vi "Vector_Plotting.vi"(1 "Template Filename":path, 2 "Data":string[][](array[string]), 3 "Channel Names":string[](array[string])) -> ()   [LabVIEW 2010]
uses:
  Data_File_Type.ctl
  Controls/Group_Binning.ctl
  Globals/Constants_global.vi
panel:
  in  "V":u16(ring) items=["LDA (UW) X Position (mm)", "LDA (UW) Y Position (mm)", "LDA (UW) Z Position (mm)", "Model Mean LDA (U)", "Model Mean LDA (W)"]
  in  "U":u16(ring) items=["LDA (UW) X Position (mm)", "LDA (UW) Y Position (mm)", "LDA (UW) Z Position (mm)", "Model Mean LDA (U)", "Model Mean LDA (W)"]
  in  "Y Axis":u16(ring) items=["LDA (UW) X Position (mm)", "LDA (UW) Y Position (mm)", "LDA (UW) Z Position (mm)", "Model Mean LDA (U)", "Model Mean LDA (W)"]
  in  "X Axis":u16(ring) items=["LDA (UW) X Position (mm)", "LDA (UW) Y Position (mm)", "LDA (UW) Z Position (mm)", "Model Mean LDA (U)", "Model Mean LDA (W)"]
  in  "OK Button":bool
  in  "Row Selector":i32(listbox)=1
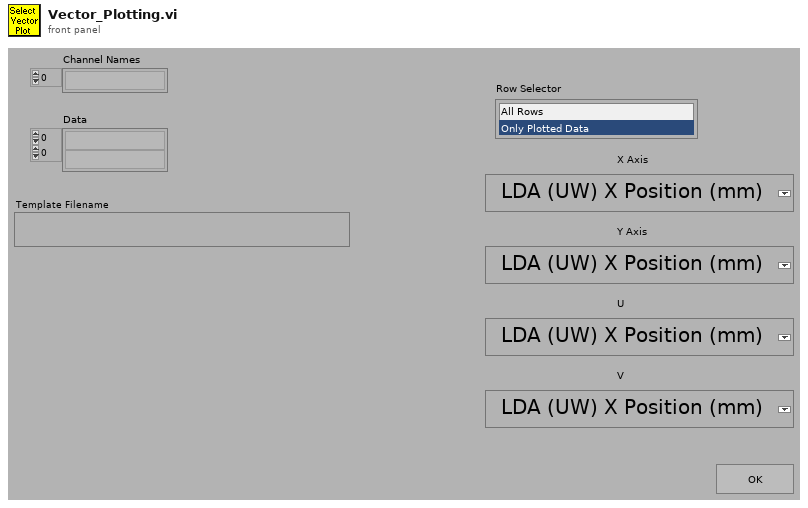
[diagram p1: front panel]
types:
  T1 = typedef "Data_File_Type.ctl" = enum16{"Read All File Types", "Results Files Only", "Raw Data Files Only", "Calibration Files Only", "Gas Desk Files Only", "Old Results Files Only", "Tabulated Data Files Only"}
  T2 = enum16{"Show only data summary", "Show data summary", "No data summary"}
  T3 = typedef "Group_Binning.ctl" = cluster{"Index":i32, "Tolerance":dbl, "Precision":string}
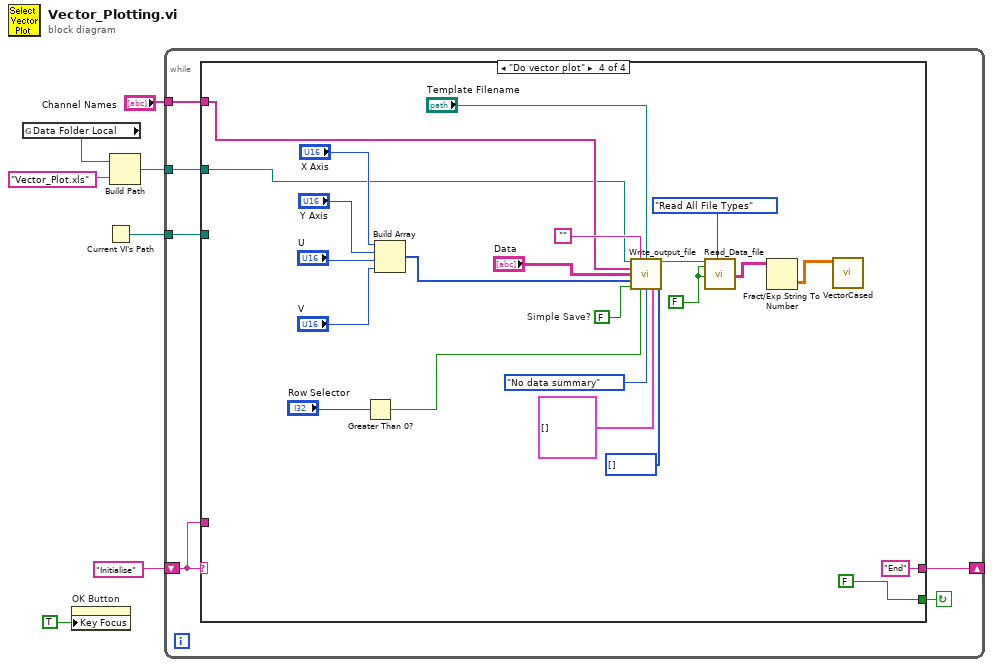
[diagram p0: block diagram]
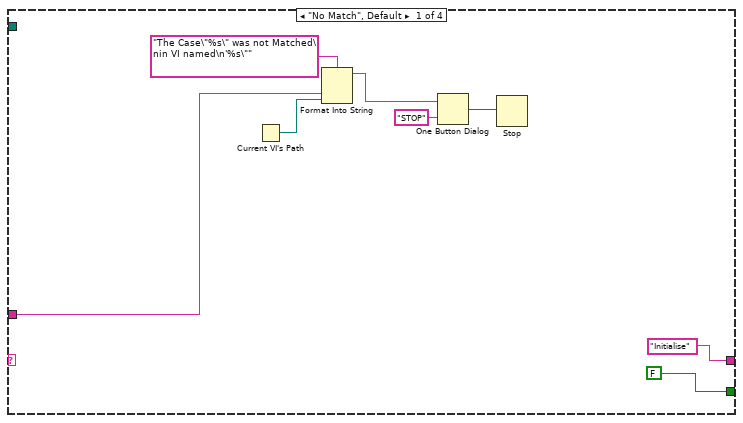
[diagram p2: hidden frame]
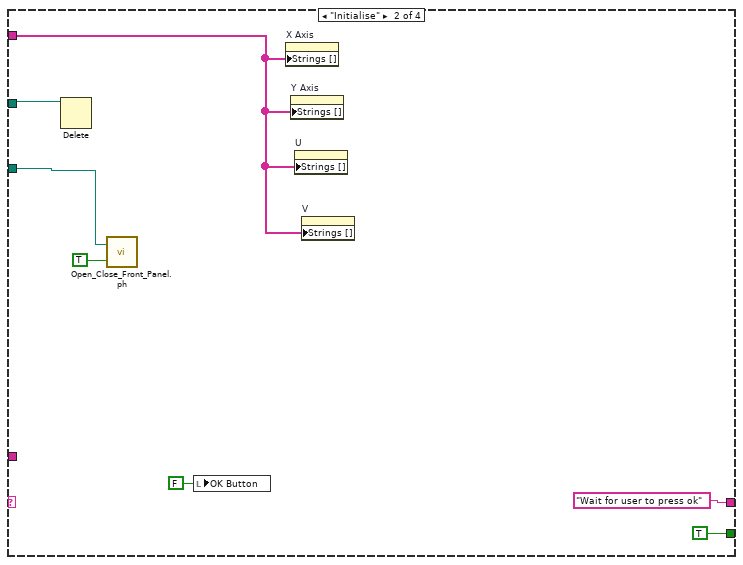
[diagram p3: hidden frame]
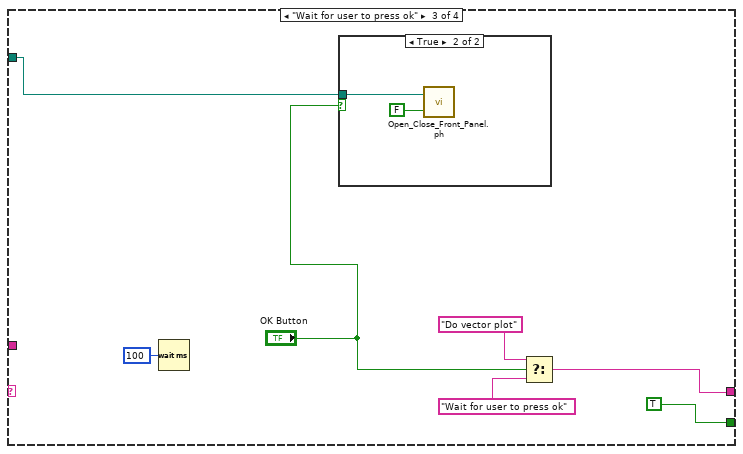
[diagram p4: hidden frame]
diagram:
  n1 = global read "Constants_global.vi" "Data Folder Local"() -> (w3:path)
  n2 = property on="OK Button" class="Bool (strict)"("Key Focus"=TRUE) -> ()  [unwired: 2 in, 2 out]
  n3 = Current VI's Path() -> (path=w6:path)
  n4 = Build Path(base path=w3, name or relative path="Vector_Plot.xls") -> (appended path=w1:path)
  n5 = while {
    shift-left: "Initialise" -> [w11]
    shift-right: [w12] -> _
    tunnel: w6 -> [w10]
    tunnel: "Channel Names" -> [w9]
    tunnel: w1 -> [w8]
    stop <- w13 continue-if-true
    n6 = case shown="\"Do vector plot\"" w11 {
      tunnel: [FALSE TRUE TRUE FALSE] -> w13
      tunnel: ["Initialise" "Wait for user to press ok" w34 "End" ("t")] -> w12
      tunnel: w11 -> [w16 _ _ _]
      tunnel: w10 -> [_ w26 w29 _]
      tunnel: w9 -> [_ w24 _ w41]
      tunnel: w8 -> [_ w22 _ w40]
      frame "No Match", Default {
        n7 = Current VI's Path() -> (path=w15:path)
        n8 = Format Into String(format string="The Case\"%s\" was not Matched\nin VI named\n'%s\"" ("Format String"), w16, w15) -> (resulting string=w19:string)  [unwired: 2 in, 1 out]
        n9 = One Button Dialog(message=w19, button name ("OK")="STOP") -> (true=w17:bool)
        n10 = Stop(stop? (T)=w17) -> ()
      }
      frame "Initialise" {
        n11 = Delete(path (use dialog)=w22) -> ()  [unwired: 1 in, 6 out]
        n12 = call "Open_Close_Front_Panel.ph.vi"("Front Panel Window:Open"=TRUE, "VI path"=w26) -> ()  [unwired: 2 out]
        n13 = local write "OK Button"(FALSE ("OK Button")) -> ()
        n14 = property on="X Axis" class="Ring (strict)"("Strings []"=w24) -> ()  [unwired: 2 in, 2 out]
        n15 = property on="Y Axis" class="Ring (strict)"("Strings []"=w24) -> ()  [unwired: 2 in, 2 out]
        n16 = property on="U" class="Ring (strict)"("Strings []"=w24) -> ()  [unwired: 2 in, 2 out]
        n17 = property on="V" class="Ring (strict)"("Strings []"=w24) -> ()  [unwired: 2 in, 2 out]
      }
      frame "Wait for user to press ok" {
        n18 = Wait (ms)(milliseconds to wait=u32 100) -> ()  [unwired: 1 out]
        n19 = case shown="True" "OK Button" {
          tunnel: w29 -> [_ w36]
          frame False {
          }
          frame True {
            n20 = call "Open_Close_Front_Panel.ph.vi"("Front Panel Window:Open"=FALSE, "VI path"=w36) -> ()  [unwired: 2 out]
          }
        }
        n21 = Select(t="Do vector plot", s="OK Button", f="Wait for user to press ok") -> (s? t:f=w34:string)
      }
      frame "Do vector plot" {
        w44 = FALSE ("Read Channel Names only")
        w53 = FALSE  # Simple Save?
        n22 = Greater Than 0?(x="Row Selector") -> (x > 0?=w54:bool)
        n23 = Build Array("X Axis", "Y Axis", "U", "V") -> (w48:u16[])
        n24 = call "Write_output_file.vi"("Output filename"=w40, "Header"="", "Template Filename"="Template Filename", "Channel Names"=w41, "Data"="Data", "Desired Columns"=w48, "Simple Save?"=w53, "Save Plotted rows only?"=w54, "Summarise mode"=T2."No data summary", "Grouping info"=T3[] [], "Channels to Tabulate in header"=i32[] []) -> ("Output filename Out"=w45:path)  [unwired: 1 in, 3 out]
        n25 = call "Read_Data_file.vi"("Results file"=w45, "Read Channel Names only"=w44, "Add Extra Channels?"=w44, "Desired File Types"=Data_File_Type."Read All File Types") -> ("Channel Values Out"=w42:string[][])  [unwired: 1 in, 14 out]
        n26 = Fract/Exp String To Number(string=w42) -> (number=w38:dbl[][])  [unwired: 4 out]
        n27 = call "VectorCased.vi"("XYUVArray"=w38) -> ()  [unwired: 11 out]
      }
    }
  }
